vi "Set scheduling.vi"(8 "error in (no error)":errorcluster, 10 "scheduling":i32, 11 "MQTT-Client in":refnum<class "MQTT-Client.lvclass">) -> (0 "error out":errorcluster, 3 "MQTT-Client out":refnum<class "MQTT-Client.lvclass">)   [LabVIEW 2023, in "MQTT-Client.lvlib" / "MQTT-Client.lvclass"]
uses:
  MQTT-Client.lvclass
  MQTT-Client.lvclass/MQTT-Client.ctl
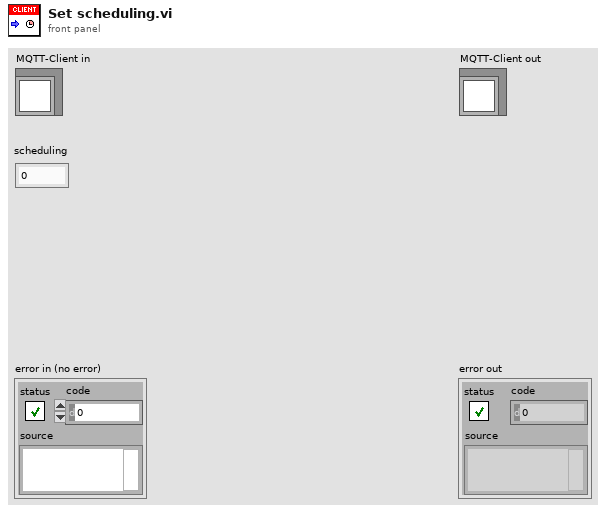
[diagram p1: front panel]
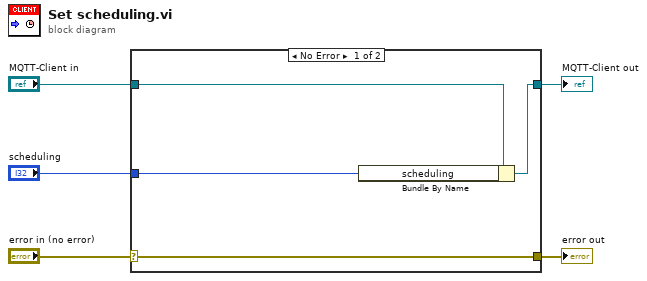
[diagram p0: block diagram]
diagram:
  n1 = case shown="No Error" "error in (no error)" {
    selector: "error in (no error)" -> [w9 w10]
    tunnel: [w9 w10] -> w4
    tunnel: [w7 w11] -> w2
    tunnel: "MQTT-Client in" -> [w8 w11]
    tunnel: "scheduling" -> [w6 _]
    frame No Error {
      n2 = Bundle By Name(cluster=w8, "scheduling"=w6) -> (w7:refnum<class "MQTT-Client.lvclass">)
    }
    frame Error {
    }
  }
  "error out" <- w4
  "MQTT-Client out" <- w2
